vi "get_subpattern.vi"(8 "error in (no error)":errorcluster, 11 "TrajectoryMH100122AODRAPS in":refnum<class "TrajectoryMH100122AODRAPS.lvclass">) -> (0 "error out":errorcluster, 1 "number of iteration points":dbl, 2 "winding number":dbl, 3 "TrajectoryMH100122AODRAPS out":refnum<class "TrajectoryMH100122AODRAPS.lvclass">, 4 "diameter":dbl, 5 "height":dbl)   [LabVIEW 2010, in "TrajectoryMH100122AODRAPS.lvclass"]
uses:
  TrajectoryMH100122AODRAPS.lvclass
  TrajectoryMH100122AODRAPS.lvclass/TrajectoryMH100122AODRAPS.ctl
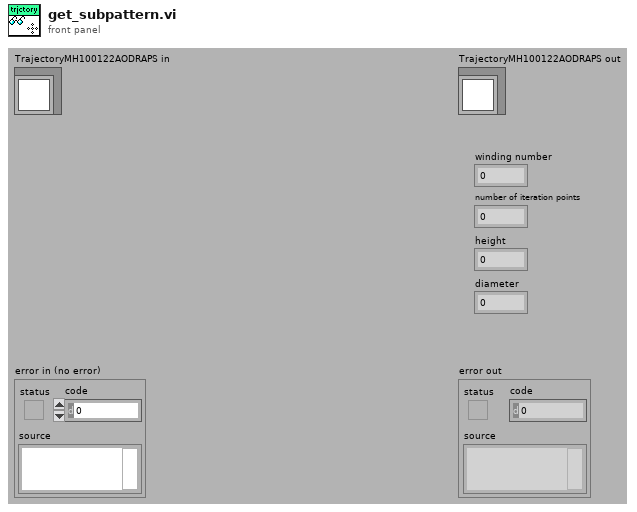
[diagram p1: front panel]
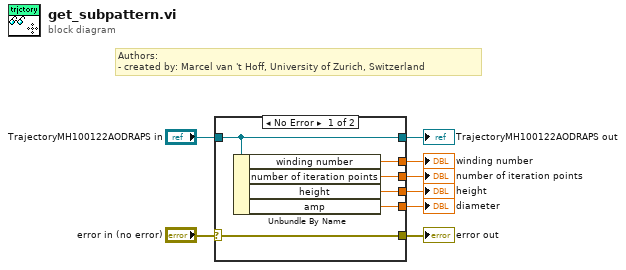
[diagram p0: block diagram]
diagram:
  # "Authors: \n- created by: Marcel van 't Hoff, University of Zurich, Switzerland"
  n1 = case shown="No Error" "error in (no error)" {
    selector: "error in (no error)" -> [w14 w16]
    tunnel: [w14 w16] -> w7
    tunnel: [w13 w15] -> w5
    tunnel: "TrajectoryMH100122AODRAPS in" -> [w13 w15]
    tunnel: [w12 _] -> w4
    tunnel: [w11 _] -> w3
    tunnel: [w10 _] -> w2
    tunnel: [w9 _] -> w1
    frame No Error {
      n2 = Unbundle By Name(w13) -> ("winding number"=w12:dbl, "number of iteration points"=w11:dbl, "height"=w10:dbl, "amp"=w9:dbl)
    }
    frame Error {
    }
  }
  "error out" <- w7
  "TrajectoryMH100122AODRAPS out" <- w5
  "winding number" <- w4
  "number of iteration points" <- w3
  "height" <- w2
  "diameter" <- w1
